vi "Complete Request.vi"(7 "Processing In":refnum<class "Processing.lvclass">, 11 "SSE Handler in":refnum<class "SSE Handler.lvclass">) -> (0 "error out":errorcluster, 5 "Processing":refnum<class "Processing.lvclass">)   [LabVIEW 2020, in "HTTP Server.lvlib" / "SSE Handler.lvclass"]
uses:
  SSE Handler.lvclass
  Processing/Processing.lvclass
  Processing/Processing.lvclass/Processing.ctl
  SSE Manager/SSE Manager.lvclass
  SSE Handler.lvclass/SSE Handler.ctl
  SSE Client/SSE Client.lvclass
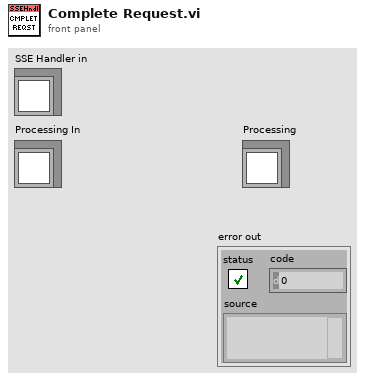
[diagram p1: front panel]
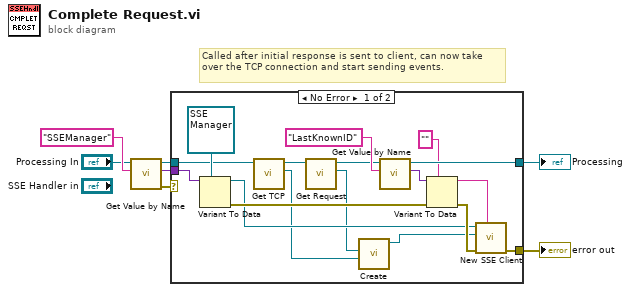
[diagram p0: block diagram]
diagram:
  # "Called after initial response is sent to client, can now take over the TCP connection and start sending events."
  n1 = call "Get Value by Name.vi"("Name"="SSEManager" ("Name for Type"), "Processing in"="Processing In") -> ("error out"=w5:errorcluster, "Value"=w4:variant, "Processing out"=w3:refnum<class "Processing.lvclass">)  [unwired: 7 in]
  n2 = case shown="No Error" w5 {
    tunnel: w4 -> [w18 _]
    tunnel: w3 -> [w15 w25]
    tunnel: [w21 w25] -> w2
    tunnel: [w8 _] -> w1
    frame No Error {
      n3 = Variant To Data(type=refnum<class "SSE Manager.lvclass"> refnum ("HTTP Server:SSE Manager.lvclass"), Variant=w18) -> (data=w16:refnum<class "SSE Manager.lvclass">, error out=w23:errorcluster)  [unwired: 1 in]
      n4 = call "Get TCP.vi"("Processing in"=w15) -> ("TCP"=w13:refnum<k5>, "Processing out"=w14:refnum<class "Processing.lvclass">)  [unwired: 9 in]
      n5 = call "Get Request.vi"("Processing in"=w14) -> ("Request"=w12:refnum<class "Request.lvclass">, "Processing out"=w11:refnum<class "Processing.lvclass">)  [unwired: 9 in]
      n6 = call "Create.vi"("TCP"=w13, "Request"=w12) -> ("SSE Client out"=w10:refnum<class "SSE Client.lvclass">)  [unwired: 8 in, 1 out]
      n7 = call "Get Value by Name.vi"("Name"="LastKnownID" ("Name for Type"), "Processing in"=w11) -> ("Value"=w20:variant, "Processing out"=w21:refnum<class "Processing.lvclass">)  [unwired: 7 in, 1 out]
      n8 = Variant To Data(error in=w23, type="", Variant=w20) -> (data=w9:string, error out=w24:errorcluster)
      n9 = call-dynamic "New SSE Client.vi"("Last Event ID (None)"=w9, "error in (no error)"=w24, "SSE Client"=w10, "SSE Manager in"=w16) -> ("error out"=w8:errorcluster)  [unwired: 6 in, 1 out]
    }
    frame Error {
      # "Not SSE connection"
    }
  }
  "error out" <- w1
  "Processing" <- w2
